vi "AlliGator Load FLI Image Folder File Information.vi"(8 "error in (no error)":errorcluster, 11 "Image Folder":path) -> (0 "error out":errorcluster, 1 "Data Description":string, 2 "Metadata":string, 3 "FLI Data File Information":T1)   [LabVIEW 2021, in "AlliGator Files.lvlib"]
doc: "Creates FLI Dataset information structure & string needed to load the dataset."
uses:
  AlliGator Files.lvlib
  AlliGator FLI Dataset Type.ctl
  AlliGator FLI Data File Information.ctl
  AlliGator HDF5.lvlib
  Files/Files.lvlib
  Image/Image.lvlib
  AlliGator RecSettings Metadata.ctl
  AlliGator Image Folder Loading Information.ctl
  AlliGator Settings.lvlib
  AlliGator Settings List.ctl
  AlliGator Load Single Gate Image from Image Folder.vi
  Phasor/Phasor Fluorescence Lifetime Parameters v3.ctl
  Phasor/Phasor.lvlib
  Variant/Variant.lvlib
panel:
  # "see the AlliGator License on the block diagram (Ctrl+E or Window:Show Block Diagram)"
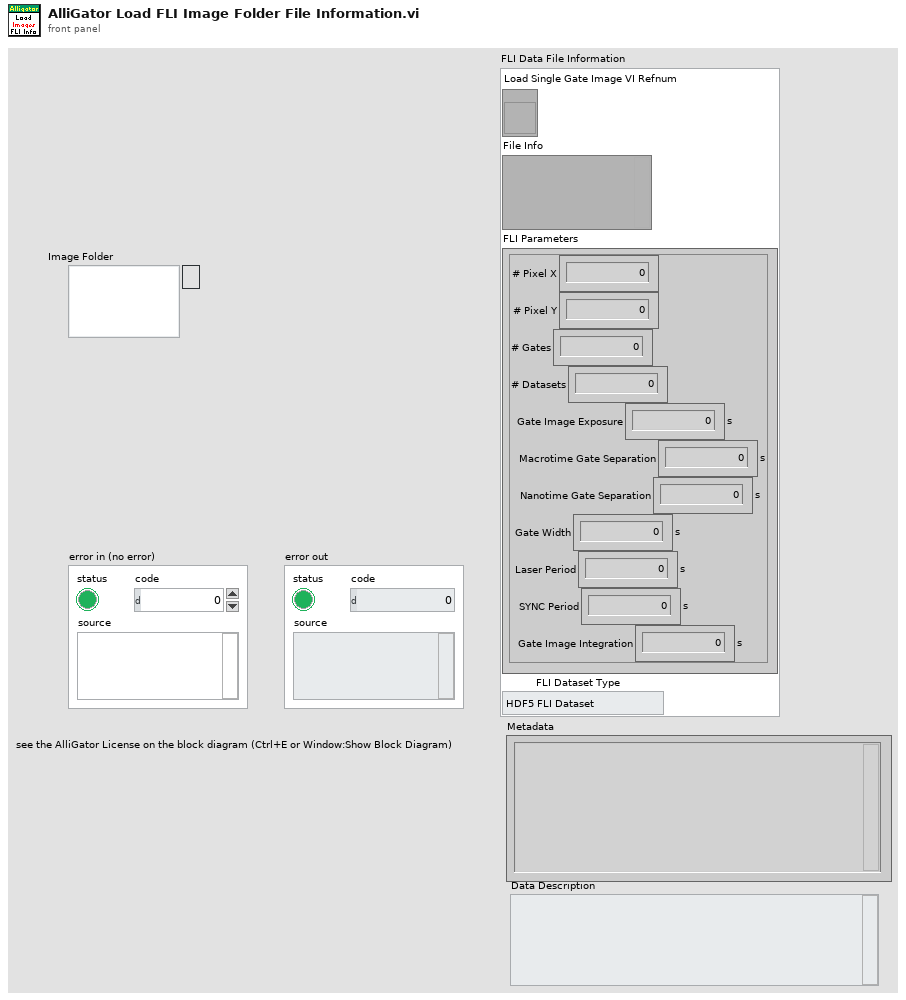
[diagram p1: front panel]
types:
  T1 = typedef "AlliGator HDF5.lvlib/AlliGator FLI Data File Information.ctl" = cluster{"Load Single Gate Image VI Refnum":refnum<vi>, "File Info":variant, "FLI Parameters":T2, "FLI Dataset Type":T3}
  T2 = typedef "Phasor.lvlib/Phasor Fluorescence Lifetime Parameters v3.ctl" = cluster{"# Pixel X":i32, "# Pixel Y":i32, "# Gates":i32, "# Datasets":i32, "Gate Image Exposure":dbl[unit], "Macrotime Gate Separation":dbl[unit], "Nanotime Gate Separation":dbl[unit], "Gate Width":dbl[unit], "Laser Period":dbl[unit], "SYNC Period":dbl[unit], "Gate Image Integration":dbl[unit]}
  T3 = typedef "AlliGator Files.lvlib/AlliGator FLI Dataset Type.ctl" = enum16{"HDF5 FLI Dataset", "Gate Image Folder", ".sdt FLI Dataset (Becker & Hickl)", ".ptu FLI Dataset (PicoQuant)", "SS1 FLI Dataset", "SS2 FLI Dataset", "I/m/phi Dataset", ".bin FLI Dataset (PicoQuant Binned)", ".bin FLI Dataset (Piccolo Binned)"}
  T4 = typedef "AlliGator Files.lvlib/AlliGator Image Folder Loading Information.ctl" = cluster{"Image Folder":path, "Metadata":T5}
  T5 = typedef "AlliGator Files.lvlib/AlliGator RecSettings Metadata.ctl" = cluster{"Time Stamp (s)":dbl, "First Gate":dbl[unit], "Gate Step":dbl[unit], "# Gates":i32, "Gate Duration":dbl[unit], "Laser Period":dbl[unit], "Gate Image Integration":dbl[unit], "Date":timestamp, "V MCP":dbl[unit], "Binning":i32}
  T6 = typedef "AlliGator Settings.lvlib/AlliGator Settings List.ctl" = enum16{"GUI:Visible Settings Tab", "GUI:Last Run Version", "Source Image:Use Image Histogram for Contrast", "Source Image:Low Count Pixels Rejection Options", "Source Image:High Count Pixels Rejection Options", "Source Image:Use Image Brightness", "Source Image:Blend Overlay with Image Background", "Source Image:Use Fixed ROI Diameter", "Source Image:ROI Diameter", "Source Image:ROI Center Color", "Source Image:Peak Threshold", "Source Image:Intensity Threshold", "Source Image:Image Binning Options", "Source Image:Image Smoothing Options", "Source Image:Image Histogram Active", "Source Image:Invert Binary Mask", "Source Image:Hot Pixel Removal", "Source Image:Overlay Analyzed ROI Center", "Source Image:Auto-Adjust Contrast", "Source Image:Histogram Lower Percentile", "Source Image:Histogram Upper Percentile", "Source Image:Save Source Image", "Source Image:Scale Bar Options", "Source Image:Image Resolution (Pixel Size)", "Source Image:Flatfield Correction", "Source Image:Show Dead Left Columns Correction", "Source Image:Dead Left Columns Correction", "Source Image:Image Pre-Processing Operations Order", "Data Information:Gate Width", "Data Information:Nanotime Gate Separation", "Data Information:Macrotime Gate Separation", "Data Information:Gate Step", "Data Information:# Gates", "Data Information:Gate Image Exposure", "Data Information:Gate Image Integration", "Data Information:Gates to Skip", "Data Information:Gates to Keep", "Data Information:Define Gates to", "Data Information:Channel Name", "Data Information:Available Channel Names", "Data Information:Channel Arithmetic", "Data Information:Background File Subtraction", "Data Information:Background File", "Data Information:Background Scaling Factor", "Data Information:Background Pile-up Correction", "Data Information:Background Pixel Well Capacity", "Data Information:Laser Period", "Data Information:SYNC Period", "Data Information:Pile-up Correction", "Data Information:Pixel Well Capacity", "Data Information:Dataset Scaling Factor", "Fluorescence Decay_Decay Pre-Processing:Reverse Gates", "Fluorescence Decay_Decay Pre-Processing:Verbose Decay Pre-Processing", "Fluorescence Decay_Decay Pre-Processing:Use Decay Pre-Processing", "Fluorescence Decay_Decay Pre-Processing:Background Subtraction", "Fluorescence Decay_Decay Pre-Processing:Background Definition Range", "Fluorescence Decay_Decay Pre-Processing:Baseline Subtraction Method", "Fluorescence Decay_Decay Pre-Processing:Decay Pre-Processing Operations Order", "Fluorescence Decay_Decay Pre-Processing:Smoothing Parameter", "Fluorescence Decay_Decay Pre-Processing:Shift Decay", "Fluorescence Decay_Decay Pre-Processing:Decay Shift Parameters", "Fluorescence Decay_Decay Pre-Processing:Fold Decay", "Fluorescence Decay_Decay Pre-Processing:# Folds", "Fluorescence Decay_Decay Pre-Processing:1-Normalize Decay", "Fluorescence Decay_Decay Pre-Processing:[0-1]-Normalize Decay", "Fluorescence Decay_Decay Pre-Processing:Smoothen Decay", "Fluorescence Decay_Decay Pre-Processing:Extrapolate Decay", "Fluorescence Decay_Decay Pre-Processing:Use Periodicity", "Fluorescence Decay_Decay Pre-Processing:Use Cursors", "Fluorescence Decay_Decay Pre-Processing:Tail Fraction", "Fluorescence Decay_Decay Pre-Processing:Head Fraction", "Fluorescence Decay_Decay Pre-Processing:Additional Points", "Fluorescence Decay_Decay Pre-Processing:Straighten Decay", "Fluorescence Decay_Decay Pre-Processing:Constant Background", "Fluorescence Decay_Decay Pre-Processing:Pixel-Normalize Decay", "Fluorescence Decay_Advanced Analysis:Extract IRF instead of Decay", "Fluorescence Decay_Advanced Analysis:IRF Extraction Options", "Fluorescence Decay_Advanced Analysis:IRF Optimization Options", "Fluorescence Decay_Advanced Analysis:Square Pulse Options", "Fluorescence Decay_Advanced Analysis:IRF Order", "Fluorescence Decay_Advanced Analysis:IRF Time Constants", "Fluorescence Decay_Advanced Analysis:Wavelet Analysis Options", "Fluorescence Decay_Advanced Analysis:Average Lifetime Options", "Fluorescence Decay_Fit Options:Fit Options", "Fluorescence Decay_Fit Options:Use Legacy Fitting Approach", "Fluorescence Decay_Fit Options:Use Data Information Laser Period", "Fluorescence Decay_Fit Parameters:Displayed Fit Parameters", "Fluorescence Decay_Fit Parameters:Fit Parameter Constraints", "Fluorescence Decay_Fit Parameters:Export Tabulated Results", "Fluorescence Decay_Fit Parameters:MLE Baseline Offset Type", "Fluorescence Decay_Fit Parameters:MLE Baseline Offset", "Fluorescence Decay_Fit Parameters:Guess Parameter Names", "Fluorescence Decay_Fit Parameters:Guess Parameter Values", "Fluorescence Decay_Fit Parameters:Guess Parameters Options", "Fluorescence Decay_Styles:Show Last Decay Only", "Fluorescence Decay_Styles:Decay Graph Color Array", "Fluorescence Decay:Decay Graph Active", "Fluorescence Decay Statistics:Min Peak Value", "Fluorescence Decay Statistics:Reject Low Decay Peak Pixels", "Fluorescence Decay Statistics:Reject High Decay Peak Pixels", "Fluorescence Decay Statistics:Max Peak Value", "Time Traces:Use File Timestamp", "Time Traces:Time Step", "Time Traces:Use Intensity Correction File", "Time Traces:Intensity Correction File", "Phasor Plot:Phasor Plot Smoothing Options", "Phasor Plot:Phasor Plot Size", "Phasor Plot:Phasor Plot Graphics Options", "Phasor Plot:Cumulative Phasor Plot", "Phasor Plot:Use Phasor Brightness", "Phasor Plot:Blend Overlay with Phasor Background", "Phasor Plot:Save Phasor Plot", "Phasor Plot:Show References", "Phasor Plot:Phasor Ratio Decay Range", "Phasor Plot:Exponential Fading", "Phasor Plot:Phasor Ratio Reference Colors", "Phasor Plot:Reference Radius", "Phasor Plot:Show Color Map Vertices", "Phasor Plot:Phasor Plot Active", "Phasor Plot:Phasor Ratio Color Map Type", "Phasor Plot:Phasor Ratio Color Map", "Phasor Plot:Phasor Ratio Display Range", "Phasor Plot:Selected Image ROI(s)", "Phasor Plot:All Image ROIs", "Phasor Plot:Selected Phasor Plot ROI(s)", "Phasor Plot:All Phasor Plot ROIs", "Phasor Plot:Phasor Ratio Color-Coded Quantity", "Phasor Plot:Store Phasor Harmonics", "Phasor Plot:Draw Reference Segment", "Phasor Plot:User-Defined Quantity", "Phasor Graph:Phasor Frequency", "Phasor Graph:Phasor Ratio Type", "Phasor Graph:Pixel-level Phasor Computation", "Phasor Graph:Save Phasor Graph", "Phasor Graph:Phasor Graph Active", "Phasor Graph:Phasor SDV Options", "Phasor Calibration:Use Backup Calibration if needed", "Phasor Graph:Define Shortest Lifetime as", "Phasor Calibration:Backup Calibration Type", "Phasor Calibration:Calibration Type", "Phasor Calibration:Calibration Lifetime", "Phasor Calibration:Calibration Map Algorithm", "Single-Exponential Phasor Locus (SEPL):Gate Parameters", "Single-Exponential Phasor Locus (SEPL):User-defined Gate", "Single-Exponential Phasor Locus (SEPL):User-defined IRF", "Single-Exponential Phasor Locus (SEPL):Phasor Parameters", "Single-Exponential Phasor Locus (SEPL):Decay & IRF Parameters", "Single-Exponential Phasor Locus (SEPL):Display Parameters", "Lifetime Analysis:Decay Analysis Parameters", "Lifetime Analysis:Lifetime Map Active", "Plugins:Python Settings", "Miscellaneous:Verbose Mode", "Miscellaneous:Beep after Script", "Miscellaneous:Saved Image File Format", "Miscellaneous:Exported Gate Image Settings", "Miscellaneous:Include Loading in Timing", "Miscellaneous:Verbose Settings Mode", "Miscellaneous:Histogram Options", "Miscellaneous:Beep on Error", "Miscellaneous:# Logical Processors Used", "Miscellaneous:ROI Description Max Characters", "Miscellaneous:Verbose Error Mode", "Miscellaneous:Transparent Mask Color"}
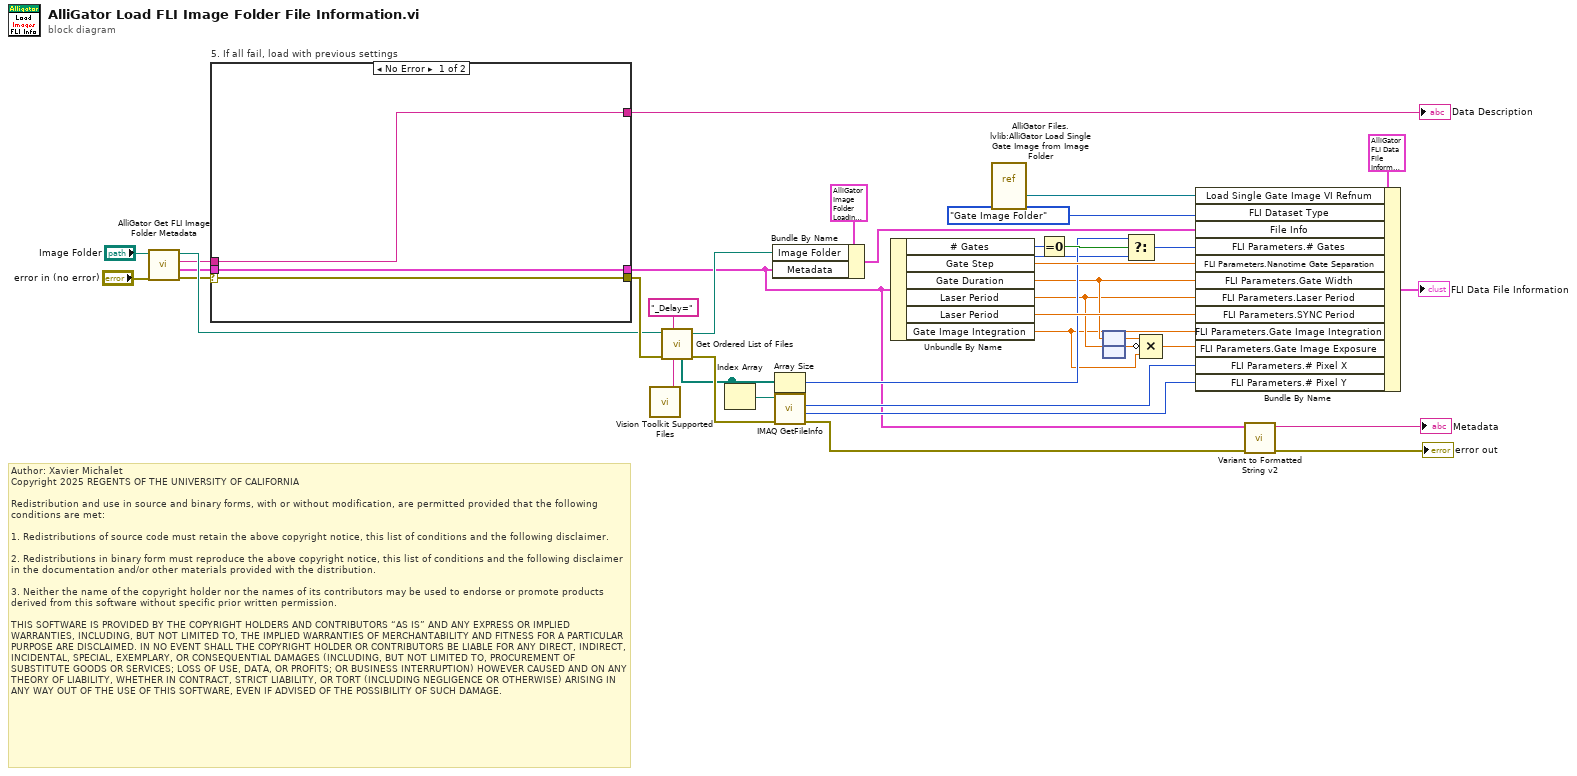
[diagram p0: block diagram]
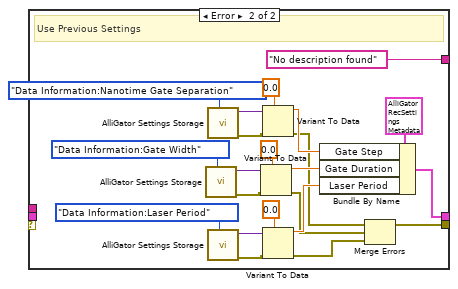
[diagram p2: hidden frame]
diagram:
  # "Author: Xavier Michalet\nCopyright 2025 REGENTS OF THE UNIVERSITY OF CALIFORNIA\n\nRedistribution and use in source and binary forms, with or without modification, are permitted provided that the following conditions are met:\n\n1. Redistributions of source code must retain the above copyright notice, this list of conditions and the following disclaimer.\n\n2. Redistributions in binary form must reproduce the above copyright notice, this list of conditions and the following disclaimer in the documentation and/or other materials provided with the distribution.\n\n3. Neither the name of the copyright holder nor the names of its contributors may be used to endorse or promote products derived from this software without specific prior written permission.\n\nTHIS SOFTWARE IS PROVIDED BY THE COPYRIGHT HOLDERS AND CONTRIBUTORS “AS IS” AND ANY EXPRESS OR IMPLIED WARRANTIES, INCLUDING, BUT NOT LIMITED TO, THE IMPLIED WARRANTIES OF MERCHANTABILITY AND FITNESS FOR A PARTICULAR PURPOSE ARE DISCLAIMED. IN NO EVENT SHALL THE COPYRIGHT HOLDER OR CONTRIBUTORS BE LIABLE FOR ANY DIRECT, INDIRECT, INCIDENTAL, SPECIAL, EXEMPLARY, OR CONSEQUENTIAL DAMAGES (INCLUDING, BUT NOT LIMITED TO, PROCUREMENT OF SUBSTITUTE GOODS OR SERVICES; LOSS OF USE, DATA, OR PROFITS; OR BUSINESS INTERRUPTION) HOWEVER CAUSED AND ON ANY THEORY OF LIABILITY, WHETHER IN CONTRACT, STRICT LIABILITY, OR TORT (INCLUDING NEGLIGENCE OR OTHERWISE) ARISING IN ANY WAY OUT OF THE USE OF THIS SOFTWARE, EVEN IF ADVISED OF THE POSSIBILITY OF SUCH DAMAGE."
  n1 = call "AlliGator Get FLI Image Folder Metadata.vi"("error in (no error)"="error in (no error)", "Image Folder in"="Image Folder") -> ("error out"=w12:errorcluster, "Metadata"=w13:T5, "Metadata String"=w14:string, "Image Folder out"=w15:path)  [unwired: 6 in]
  n2 = case "5. If all fail, load with previous settings" shown="No Error" w12 {
    selector: w12 -> [w41 _]
    tunnel: [w41 w44] -> w22
    tunnel: w13 -> [w40 _]
    tunnel: [w40 w46] -> w4
    tunnel: w14 -> [w39 _]
    tunnel: [w39 "No description found" ("Settings String")] -> w21
    frame No Error {
    }
    frame Error {
      # "Use Previous Settings"
      n3 = call "AlliGator Settings Storage.vi"("AlliGator Settings List"=AlliGator_Settings_List."Data Information:Gate Width") -> ("Error Out"=w55:errorcluster, "Variant Data out"=w54:variant)  [unwired: 9 in]
      n4 = call "AlliGator Settings Storage.vi"("AlliGator Settings List"=AlliGator_Settings_List."Data Information:Nanotime Gate Separation") -> ("Error Out"=w59:errorcluster, "Variant Data out"=w60:variant)  [unwired: 9 in]
      n5 = call "AlliGator Settings Storage.vi"("AlliGator Settings List"=AlliGator_Settings_List."Data Information:Laser Period") -> ("Error Out"=w50:errorcluster, "Variant Data out"=w51:variant)  [unwired: 9 in]
      n6 = Variant To Data(error in=w55, type=dbl[unit] 0.0 ("Gate Step"), Variant=w54) -> (data=w48:dbl[unit], error out=w43:errorcluster)
      n7 = Variant To Data(error in=w59, type=dbl[unit] 0.0 ("Gate Step"), Variant=w60) -> (data=w57:dbl[unit], error out=w42:errorcluster)
      n8 = Variant To Data(error in=w50, type=dbl[unit] 0.0 ("Gate Step"), Variant=w51) -> (data=w47:dbl[unit], error out=w45:errorcluster)
      n9 = Bundle By Name(cluster=T5 {"Time Stamp (s)"=0.0, "First Gate"=0.0, "Gate Step"=0.0, "# Gates"=0, "Gate Duration"=0.0, "Laser Period"=0.0, "Gate Image Integration"=0.0, "Date"=timestamp(0 s since 1904-01-01), "V MCP"=0.0, "Binning"=0} ("Metadata"), "Gate Step"=w57, "Gate Duration"=w48, "Laser Period"=w47) -> (w46:T5)
      n10 = Merge Errors(w42, w43, w45) -> (w44:errorcluster)
    }
  }
  "Data Description" <- w21
  n11 = call "Vision Toolkit Supported Files.vi"() -> ("Pattern String"=w27:string)  [unwired: 7 in, 1 out]
  n12 = call "Get Ordered List of Files.vi"("pattern"=w27, "Split string"="_Delay=", "Error In"=w22, "Folder Path"=w15) -> ("Error Out"=w33:errorcluster, "Folder Path dup"=w24:path, "Ordered File Paths"=w18:path[])  [unwired: 4 in, 1 out]
  n13 = Index Array(array=w18) -> (element=w32:path)  [unwired: 1 in]
  n14 = Bundle By Name(cluster=T4 {"Image Folder"=path "", "Metadata"={"Time Stamp (s)"=0.0, "First Gate"=0.0, "Gate Step"=0.0, "# Gates"=0, "Gate Duration"=0.0, "Laser Period"=0.0, "Gate Image Integration"=0.0, "Date"=timestamp(0 s since 1904-01-01), "V MCP"=0.0, "Binning"=0}} ("Image Folder Loading Information"), "Image Folder"=w24, "Metadata"=w4) -> (w23:T4)
  n15 = Array Size(array=w18) -> (size(s)=w17:i32)
  n16 = call "IMAQ GetFileInfo"("error in (no error)"=w33, "File Path"=w32) -> ("error out"=w3:errorcluster, "Y Resolution"=w30:i32, "X Resolution"=w31:i32)  [unwired: 3 in, 4 out]
  n17 = Unbundle By Name(w4) -> ("# Gates"=w16:i32, "Gate Step"=w29:dbl[unit], "Gate Duration"=w10:dbl[unit], "Laser Period"=w8:dbl[unit], "Laser Period"=w28:dbl[unit], "Gate Image Integration"=w6:dbl[unit])
  n18 = vi-ref "AlliGator Files.lvlib:AlliGator Load Single Gate Image from Image Folder.vi"() -> (w35:refnum<vi>)
  n19 = Equal To 0?(x=w16) -> (x = 0?=w20:bool)
  n20 = node(w10) -> (w9:dbl)
  n21 = node(w8) -> (w7:dbl)
  n22 = Select(t=w17, s=w20, f=w16) -> (s? t:f=w19:i32)
  n23 = Compound Arithmetic op=MULTIPLY(w9, invert w7, w6) -> (w5:dbl[unit])
  n24 = Bundle By Name(cluster=T1 {"Load Single Gate Image VI Refnum"=refnum, "File Info"=variant, "FLI Parameters"={"# Pixel X"=0, "# Pixel Y"=0, "# Gates"=0, "# Datasets"=0, "Gate Image Exposure"=0.0, "Macrotime Gate Separation"=0.0, "Nanotime Gate Separation"=0.0, "Gate Width"=0.0, "Laser Period"=0.0, "SYNC Period"=0.0, "Gate Image Integration"=0.0}, "FLI Dataset Type"=enum."HDF5 FLI Dataset"} ("FLI Data File Information"), "Load Single Gate Image VI Refnum"=w35, "FLI Dataset Type"=AlliGator_FLI_Dataset_Type."Gate Image Folder", "File Info"=w23, "FLI Parameters.# Gates"=w19, "FLI Parameters.Nanotime Gate Separation"=w29, "FLI Parameters.Gate Width"=w10, "FLI Parameters.Laser Period"=w8, "FLI Parameters.SYNC Period"=w28, "FLI Parameters.Gate Image Integration"=w6, "FLI Parameters.Gate Image Exposure"=w5, "FLI Parameters.# Pixel X"=w31, "FLI Parameters.# Pixel Y"=w30) -> (→"FLI Data File Information":T1)
  n25 = call "Variant to Formatted String v2.vi"("error in (no error)"=w3, "Anything"=w4) -> ("error out"=→"error out":errorcluster, "String"=→"Metadata":string)  [unwired: 8 in]
